vi "Initialize ErrorHandling Attribute.vi"(7 "Attribute.ErrorHandling in":refnum<class "Attribute.ErrorHandling.lvclass">, 11 "Shutdown on Unhandled Error":bool) -> (3 "Attribute.ErrorHandling":refnum<class "Attribute.ErrorHandling.lvclass">)   [LabVIEW 2013, in "Attribute.ErrorHandling.lvclass"]
uses:
  Attribute.ErrorHandling.lvclass
  Definitions/def.SMO/Scope -- Enum.ctl
  Attribute/Attribute.lvclass/Attribute.ctl
  Attribute.ErrorHandling.lvclass/Attribute.ErrorHandling.ctl
  Definitions/def.SMO/def.SMO.lvclass
  Attribute/Attribute.lvclass
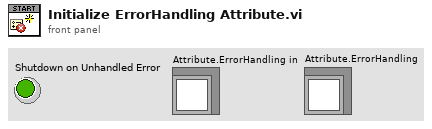
[diagram p1: front panel]
types:
  T1 = typedef "def.SMO.lvclass/Scope -- Enum.ctl" = enum16{"Public", "Protected", "Private"}
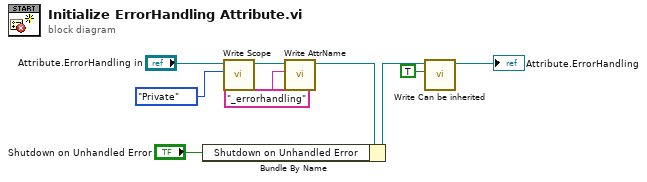
[diagram p0: block diagram]
diagram:
  n1 = call "Write Scope.vi"("Scope"=Scope_--_Enum."Private", "Attribute in"="Attribute.ErrorHandling in") -> ("Attribute out"=w8:refnum<class "Attribute.ErrorHandling.lvclass">)  [unwired: 9 in]
  n2 = call "Write AttrName.vi"("Attribute Name"="_errorhandling", "Attribute in"=w8) -> ("Attribute out"=w7:refnum<class "Attribute.ErrorHandling.lvclass">)  [unwired: 9 in]
  n3 = Bundle By Name(cluster=w7, "Shutdown on Unhandled Error"="Shutdown on Unhandled Error") -> (w3:refnum<class "Attribute.ErrorHandling.lvclass">)
  n4 = call "Write Can be inherited.vi"("Can be inherited"=TRUE, "Attribute in"=w3) -> ("Attribute out"=→"Attribute.ErrorHandling":refnum<class "Attribute.ErrorHandling.lvclass">)  [unwired: 8 in, 1 out]
